vi "Serial Read for Arduino with Control - timer.vi"() -> ()   [LabVIEW 2024]
doc: "This example performs writes and reads on a serial port, as directed by the user. You can press the Write and Read buttons, and change the Read Count, while the example is running.\n\nThe parameters set for the serial port must match the parameters of the connected instrument or device. In this example, the Read Count parameter specifies the number of bytes that the serial port reads. If there were more bytes at the port than the specified number, those bytes would not be read. If there were less bytes at the port than the specified number, you would receive a timeout error.\n\nThis example expands upon the flow control options for XON and XOFF, allowing the user to choose those control characters. Also, the user can enable or disable a termination character. Some devices require a termination character in order to identify the end of command strings. Some devices send a termination character to signify the end of data to be read. This example shows how you can end the Read operation once a termination character is detected in the buffer and/or append a termination character at the end of the Write data."
uses:
  support/Serial - Settings.ctl
  <vilib>/Instr/_visa.llb/VISA Flush IO Buffer Mask.ctl
  <vilib>/Instr/_visa.llb/VISA Configure Serial Port (Instr).vi
panel:
  out "Froce Chart":dbl[][](graph)
  out "Past Time(Sec)":dbl
  out "Cantilever Chart":dbl[][](graph)
  in  "dt for Sampling (600Hz)":dbl=0.00166
  out "Filename Out":path
  out "Data Writing":bool caption="Saving Data"
  in  "Data Format":enum32{"Foece Mode", "Raw Mode"}(radio)=enum."Raw Mode"
  in  "Zero Reset":bool
  in  "Termination Character":u8=10 format="%.0x"
  in  "End Write on \nTermination Character?":bool=TRUE
  in  "Stop Measurment":bool
  in  "Serial Settings":T1={"baud rate"=115200, "data bits"=8, "parity"=enum."None", "stop bits"=10, "flow control"=0} {"flow control" items=["None"=0, "XON/XOFF"=1, "RTS/CTS"=2, "DTR/DSR"=4]; "stop bits" items=["1.0"=10, "1.5"=15, "2.0"=20]; "data bits" min=5 max=8 step=1; "baud rate" items=["75"=75, "110"=110, "134"=134, "150"=150, "300"=300, "600"=600, "1200"=1200, "1800"=1800, "2400"=2400, "4800"=4800, "7200"=7200, "9600"=9600, "14400"=14400, "19200"=19200, "28800"=28800, "38400"=38400, "56000"=56000, "57600"=57600, "115200"=115200, "128000"=128000, "230400"=230400]}
  in  "End Read on \nTermination Character?":bool=TRUE
  in  "VISA resource name":refnum<visa-resource-name>="COM1"
  # "Overview: Serial Based Data Viewer\n\nBefore Start VI \n1: Set Serial Port as Arduino Prot\n2: Select data format ( Force or Cantilever Raw)\n3: Start VI"
  # "While Operation\n1: VI asks save measirement on file as LVM format\n    If you do not need save, just cacel the dialog.\n2: If you need to switch data mode, just clock    Force or Raw.\n3: If you need to reset offcet, click zero offset."
  # "Ver 18.Jun.2024.b\nThis LV was made by Haruo Noma\non 01/Jun/2024\n\nYou can copy & modify as you like \nHoever, no responsibility for using this LV."
  # "0xA is equivalent to a '\\n' character, which is a line feed."
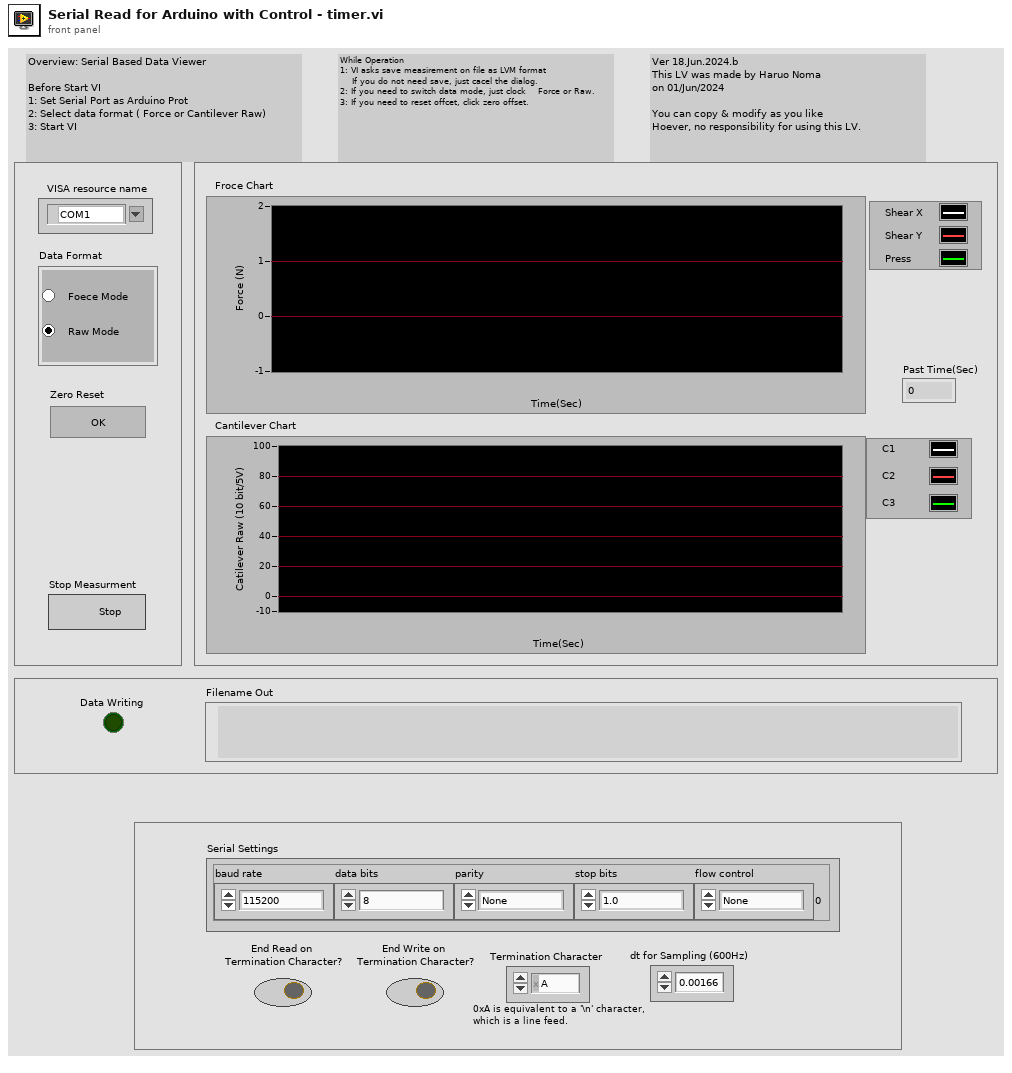
[diagram p1: front panel]
types:
  T1 = typedef "Serial - Settings.ctl" = cluster{"baud rate":u32, "data bits":u16, "parity":enum16{"None", "Odd", "Even", "Mark", "Space"}, "stop bits":u16, "flow control":u16}
  T2 = typedef "VISA Flush IO Buffer Mask.ctl" = u16
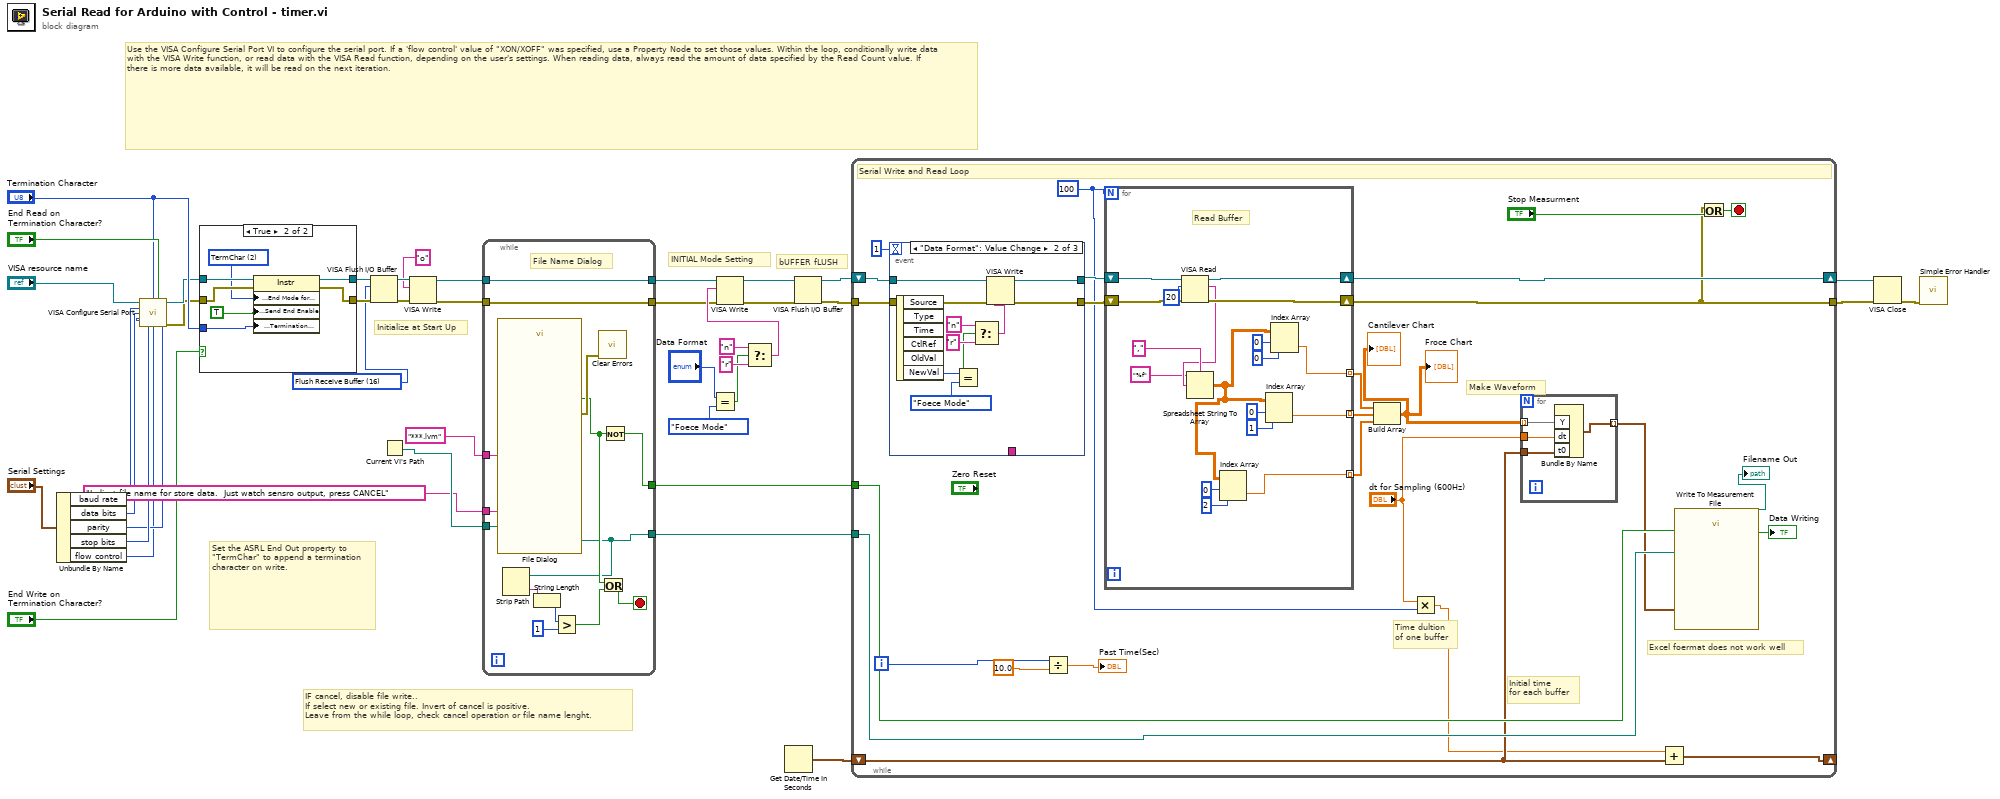
[diagram p0: block diagram]
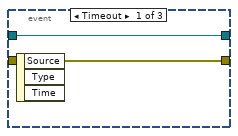
[diagram p3: hidden frame]
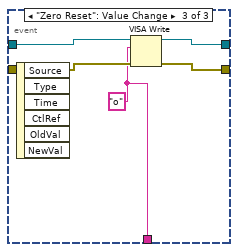
[diagram p4: hidden frame]
diagram:
  w25 = T2 16 items=["Flush Receive Buffer"=16, "Write Transmit Buffer to Device"=32, "Flush Receive Buffer (No I/O)"=64, "Flush Transmit Buffer"=128] ("Mask")
  # "bUFFER fLUSH"
  # "INITIAL Mode Setting"
  # "IF cancel, disable file write..\nIf select new or existing file. Invert of cancel is positive.\nLeave from the while loop, check cancel operation or file name lenght."
  # "Initialize at Start Up"
  # "Set the ASRL End Out property to \"TermChar\" to append a termination character on write."
  # "Use the VISA Configure Serial Port VI to configure the serial port. If a 'flow control' value of \"XON/XOFF\" was specified, use a Property Node to set those values. Within the loop, conditionally write data with the VISA Write function, or read data with the VISA Read function, depending on the user's settings. When reading data, always read the amount of data specified by the Read Count value. If there is more data available, it will be read on the next iteration."
  n1 = Unbundle By Name("Serial Settings") -> ("baud rate"=w37:u32, "data bits"=w38:u16, "parity"=w39:enum16{"None", "Odd", "Even", "Mark", "Space"}, "stop bits"=w40:u16, "flow control"=w34:u16)
  n2 = call-poly "VISA Configure Serial Port"("VISA resource name"="VISA resource name", "termination char\n(0xA = '\\n' = LF)"="Termination Character", "Enable Termination\nChar (T)"="End Read on \nTermination Character?", "baud rate (9600)"=w37, "data bits (8)"=w38, "parity (0:none)"=w39, "stop bits (10: 1 bit)"=w40, "flow control (0:none)"=w34) -> ("VISA resource name out"=w31:refnum<visa-resource-name>, "error out"=w30:errorcluster)  [unwired: 2 in, 4 out]
  n3 = case shown="True" "End Write on \nTermination Character?" {
    tunnel: w31 -> [w42 w50]
    tunnel: w30 -> [w43 w49]
    tunnel: [w42 w48] -> w27
    tunnel: [w43 w47] -> w26
    tunnel: "Termination Character" -> [_ w45]
    frame False {
    }
    frame True {
      w46 = u16 2 items=["None", "LastBit", "TermChar", "Break"] ("Serial Settings:Serial End Mode for Writes")
      n4 = property class="Instr"(reference=w50, error in=w49, "Serial Settings:End Mode for Writes"=w46, "Message Based Settings:Send End Enable"=TRUE, "Message Based Settings:Termination Character"=w45) -> (reference out=w48:refnum<visa-resource-name>, error out=w47:errorcluster)
    }
  }
  n5 = VISA Flush I/O Buffer(VISA resource name=w27, mask (16)=w25, error in (no error)=w26) -> (VISA resource name out=w24:refnum<visa-resource-name>, error out=w23:errorcluster)
  n6 = Current VI's Path() -> (path=w19:path)
  n7 = VISA Write(VISA resource name=w24, write buffer="o", error in (no error)=w23) -> (VISA resource name out=w7:refnum<visa-resource-name>, error out=w6:errorcluster)  [unwired: 1 out]
  n8 = while {
    tunnel: [w64] -> w13
    tunnel: w7 -> [w64]
    tunnel: [w63] -> w12
    tunnel: w6 -> [w63]
    tunnel: [w55] -> w21
    tunnel: [w61] -> w20
    tunnel: w19 -> [w60]
    tunnel: "Indicat file name for store data.  Just watch sensro output, press CANCEL" ("prompt") -> [w57]
    tunnel: "***.lvm" ("default name") -> [w51]
    stop <- w58 stop-if-true
    # "File Name Dialog"
    n9 = call "File Dialog"("start path"=w60, "prompt"=w57, "default name"=w51) -> ("selected path"=w55:path, "cancelled"=w59:bool, "error out"=w62:errorcluster)  [unwired: 9 in, 1 out]
    n10 = Strip Path(path=w55) -> (name=w56:string)  [unwired: 1 out]
    n11 = String Length(string=w56) -> (length=w54:i32)
    n12 = Greater?(x=w54, y=1) -> (0:w52:bool)
    n13 = call <vilib>:"Clear Errors.vi"("error in (no error)"=w62) -> ()  [unwired: 5 in, 2 out]
    n14 = Or(x=w59, y=w52) -> (x .or. y?=w58:bool)
    n15 = Not(x=w59) -> (.not. x?=w61:bool)
  }
  n16 = Equal?(x="Data Format", y=enum16{"Foece Mode", "Raw Mode", ""}."Foece Mode") -> (x = y?=w10:bool)
  n17 = Select(t="n", s=w10, f="r") -> (s? t:f=w14:string)
  n18 = VISA Write(VISA resource name=w13, write buffer=w14, error in (no error)=w12) -> (VISA resource name out=w5:refnum<visa-resource-name>, error out=w3:errorcluster)  [unwired: 1 out]
  n19 = Get Date/Time In Seconds() -> (seconds since 1Jan1904=w8:timestamp)
  n20 = VISA Flush I/O Buffer(VISA resource name=w5, error in (no error)=w3) -> (VISA resource name out=w4:refnum<visa-resource-name>, error out=w2:errorcluster)  [unwired: 1 in]
  n21 = while {
    shift-right: [w88] -> w1
    shift-left: w4 -> [w85]
    tunnel: w2 -> [w86]
    tunnel: [w87] -> w29
    tunnel: w21 -> [w75]
    tunnel: w20 -> [w74]
    shift-right: [w73] -> _
    shift-left: w8 -> [w72]
    i -> [w77]
    stop <- w90 stop-if-true
    w71 = 100
    # "Initial time \nfor each buffer"
    # "Time dultion\nof one buffer"
    # "Excel foermat does not work well"
    # "Make Waveform"
    # "Serial Write and Read Loop"
    n22 = event shown="[1] \"Data Format\": Value Change" {
      selector: _ -> [_ _ _]
      dyn-events: _ -> [_ _ _]
      timeout: 1 -> [_ _ _]
      tunnel: w86 -> [w95 w105 w111]
      tunnel: w85 -> [w96 w106 w110]
      tunnel: [w96 w103 w109] -> w84
      tunnel: [w95 w104 w108] -> w83
      tunnel: [_ _ w107] -> _
      event Timeout {
        n23 = event-data() -> ()  [unwired: 1 in, 3 out]
      }
      event "Data Format": Value Change {
        n24 = event-data() -> ("NewVal"=w101:enum32{"Foece Mode", "Raw Mode"})  [unwired: 1 in, 5 out]
        n25 = Equal?(x=w101, y=enum16{"Foece Mode", "Raw Mode", ""}."Foece Mode") -> (x = y?=w98:bool)
        n26 = Select(t="n", s=w98, f="r") -> (s? t:f=w97:string)
        n27 = VISA Write(VISA resource name=w106, write buffer=w97, error in (no error)=w105) -> (VISA resource name out=w103:refnum<visa-resource-name>, error out=w104:errorcluster)  [unwired: 1 out]
      }
      event "Zero Reset": Value Change {
        w107 = "o" ("write buffer")
        n28 = event-data() -> ()  [unwired: 1 in, 6 out]
        n29 = VISA Write(VISA resource name=w110, write buffer=w107, error in (no error)=w111) -> (VISA resource name out=w109:refnum<visa-resource-name>, error out=w108:errorcluster)  [unwired: 1 out]
      }
    }
    n30 = Divide(x=w77, y=10.0 ("x")) -> (x/y=→"Past Time(Sec)":dbl)
    n31 = for {
      N: w71 -> [_]
      shift-right: [w126] -> w88
      shift-left: w84 -> [w129]
      shift-right: [w127] -> w87
      shift-left: w83 -> [w128]
      tunnel: [w118] -> w67 mode=indexing
      tunnel: [w117] -> w66 mode=indexing
      tunnel: [w113] -> w68 mode=indexing
      # "Read Buffer"
      n32 = VISA Read(VISA resource name=w129, byte count=u32 20, error in (no error)=w128) -> (VISA resource name out=w126:refnum<visa-resource-name>, read buffer=w120:string, error out=w127:errorcluster)  [unwired: 1 out]
      n33 = Spreadsheet String To Array(delimiter (Tab)=",", format string="%f", spreadsheet string=w120) -> (array=w114:dbl[][])  [unwired: 1 in]
      n34 = Index Array(array=w114, index (row)=0, index (col)=2 ("disabled index (col)")) -> (element=w113:dbl)
      n35 = Index Array(array=w114, index (row)=0, index (col)=1 ("disabled index (col)")) -> (element=w118:dbl)
      n36 = Index Array(array=w114, index (row)=0, index (col)=0 ("disabled index (col)")) -> (element=w117:dbl)
    }
    n37 = Build Array(w66, w67, w68) -> (w79:dbl[][])
    "Cantilever Chart" <- w79
    "Froce Chart" <- w79
    n38 = Multiply(x="dt for Sampling (600Hz)", y=w71) -> (x*y=w69:dbl)
    n39 = for {
      tunnel: w79 -> [w92] mode=indexing
      tunnel: [w94] -> w65 mode=indexing
      tunnel: "dt for Sampling (600Hz)" -> [w93]
      tunnel: w72 -> [w91]
      n40 = Bundle By Name("Y"=w92, "dt"=w93, "t0"=w91) -> (w94:waveform(dbl))  [unwired: 1 in]
    }
    n41 = Add(x=w69, y=w72) -> (x+y=w73:timestamp)
    n42 = call "Write To Measurement File"("Signals"=w65, "Enable"=w74, "Filename"=w75) -> ("Filename Out"=→"Filename Out":path, "Saving Data"=→"Data Writing":bool)  [unwired: 14 in, 1 out]
    n43 = Or(x=w87, y="Stop Measurment") -> (x .or. y?=w90:bool)
  }
  n44 = VISA Close(VISA resource name=w1, error in (no error)=w29) -> (error out=w28:errorcluster)
  n45 = call <vilib>:"Simple Error Handler.vi"("error in (no error)"=w28) -> ()  [unwired: 1 in, 8 out]
